vi "Shock&Dyanamics Laboratory - DROPBEAR_June2022_Rev3.vi"() -> ()   [LabVIEW 2019] (continued)
                    n420 = property on="PF Card 29" class="DigNum (strict)"(error in=w420, "DisabledEnum"=w419) -> (error out=w421:errorcluster)  [unwired: 1 in, 1 out]
                    n421 = property on="PF Channel 29" class="DigNum (strict)"(error in=w421, "DisabledEnum"=w419) -> (error out=w422:errorcluster)  [unwired: 1 in, 1 out]
                  }
                  frame True {
                    n422 = stacked-sequence {
                      tunnel: [w427 _] -> w424
                      frame #0 {
                        n423 = property on="PF Condition 29" class="Bool (strict)"() -> (error out=w430:errorcluster, "Value"=w425:bool)  [unwired: 2 in, 1 out]
                        n424 = case shown="True" w425 {
                          tunnel: [T42."Disabled and Grayed Out" ("Disabled") T42."Enabled" ("Disabled")] -> w426
                          frame False {
                          }
                          frame True {
                          }
                        }
                        n425 = property on="PF Chassis 29" class="DigNum (strict)"(error in=w430, "DisabledEnum"=w426) -> (error out=w429:errorcluster)  [unwired: 1 in, 1 out]
                        n426 = property on="PF Card 29" class="DigNum (strict)"(error in=w429, "DisabledEnum"=w426) -> (error out=w428:errorcluster)  [unwired: 1 in, 1 out]
                        n427 = property on="PF Channel 29" class="DigNum (strict)"(error in=w428, "DisabledEnum"=w426) -> (error out=w427:errorcluster)  [unwired: 1 in, 1 out]
                      }
                      frame #1 {
                        n428 = property on="Signal Type 29" class="Enum (strict)"() -> (error out=w435:errorcluster, "Value"=w436:T8)  [unwired: 2 in, 1 out]
                        n429 = case shown="\"Voltage\", Default" w436 {
                          tunnel: [T42."Enabled" ("Disabled") T42."Disabled and Grayed Out" ("Disabled")] -> w434
                          frame "Strain" {
                          }
                          frame "Voltage", Default {
                          }
                        }
                        n430 = property on="SG Pair 29" class="Bool (strict)"(error in=w435, "DisabledEnum"=w434) -> (error out=w433:errorcluster)  [unwired: 1 in, 1 out]
                        n431 = property on="SG Pair Ch 29" class="Enum (strict)"(error in=w433, "DisabledEnum"=w434) -> ()  [unwired: 1 in, 2 out]
                      }
                    }
                  }
                }
                n432 = case shown="False" w208 {
                  tunnel: [w573 T42."Enabled" ("Disabled")] -> w126
                  tunnel: [w576 w577] -> w151
                  frame False {
                    w573 = T42."Disabled and Grayed Out" ("Disabled")
                    n433 = property on="SG Pair 22" class="Bool (strict)"("DisabledEnum"=w573) -> (error out=w572:errorcluster)  [unwired: 2 in, 1 out]
                    n434 = property on="SG Pair Ch 22" class="Enum (strict)"(error in=w572, "DisabledEnum"=w573) -> (error out=w571:errorcluster)  [unwired: 1 in, 1 out]
                    n435 = property on="PF Chassis 22" class="DigNum (strict)"(error in=w571, "DisabledEnum"=w573) -> (error out=w574:errorcluster)  [unwired: 1 in, 1 out]
                    n436 = property on="PF Card 22" class="DigNum (strict)"(error in=w574, "DisabledEnum"=w573) -> (error out=w575:errorcluster)  [unwired: 1 in, 1 out]
                    n437 = property on="PF Channel 22" class="DigNum (strict)"(error in=w575, "DisabledEnum"=w573) -> (error out=w576:errorcluster)  [unwired: 1 in, 1 out]
                  }
                  frame True {
                    n438 = stacked-sequence {
                      tunnel: [w583 _] -> w577
                      frame #0 {
                        n439 = property on="PF Condition 22" class="Bool (strict)"() -> (error out=w580:errorcluster, "Value"=w584:bool)  [unwired: 2 in, 1 out]
                        n440 = case shown="True" w584 {
                          tunnel: [T42."Disabled and Grayed Out" ("Disabled") T42."Enabled" ("Disabled")] -> w579
                          frame False {
                          }
                          frame True {
                          }
                        }
                        n441 = property on="PF Chassis 22" class="DigNum (strict)"(error in=w580, "DisabledEnum"=w579) -> (error out=w581:errorcluster)  [unwired: 1 in, 1 out]
                        n442 = property on="PF Card 22" class="DigNum (strict)"(error in=w581, "DisabledEnum"=w579) -> (error out=w582:errorcluster)  [unwired: 1 in, 1 out]
                        n443 = property on="PF Channel 22" class="DigNum (strict)"(error in=w582, "DisabledEnum"=w579) -> (error out=w583:errorcluster)  [unwired: 1 in, 1 out]
                      }
                      frame #1 {
                        n444 = property on="Signal Type 22" class="Enum (strict)"() -> (error out=w589:errorcluster, "Value"=w590:T8)  [unwired: 2 in, 1 out]
                        n445 = case shown="\"Voltage\", Default" w590 {
                          tunnel: [T42."Enabled" ("Disabled") T42."Disabled and Grayed Out" ("Disabled")] -> w588
                          frame "Strain" {
                          }
                          frame "Voltage", Default {
                          }
                        }
                        n446 = property on="SG Pair 22" class="Bool (strict)"(error in=w589, "DisabledEnum"=w588) -> (error out=w587:errorcluster)  [unwired: 1 in, 1 out]
                        n447 = property on="SG Pair Ch 22" class="Enum (strict)"(error in=w587, "DisabledEnum"=w588) -> ()  [unwired: 1 in, 2 out]
                      }
                    }
                  }
                }
                n448 = case shown="False" w206 {
                  tunnel: [w529 T42."Enabled" ("Disabled")] -> w124
                  tunnel: [w532 w533] -> w135
                  frame False {
                    w529 = T42."Disabled and Grayed Out" ("Disabled")
                    n449 = property on="SG Pair 24" class="Bool (strict)"("DisabledEnum"=w529) -> (error out=w528:errorcluster)  [unwired: 2 in, 1 out]
                    n450 = property on="SG Pair Ch 24" class="Enum (strict)"(error in=w528, "DisabledEnum"=w529) -> (error out=w527:errorcluster)  [unwired: 1 in, 1 out]
                    n451 = property on="PF Chassis 24" class="DigNum (strict)"(error in=w527, "DisabledEnum"=w529) -> (error out=w530:errorcluster)  [unwired: 1 in, 1 out]
                    n452 = property on="PF Card 24" class="DigNum (strict)"(error in=w530, "DisabledEnum"=w529) -> (error out=w531:errorcluster)  [unwired: 1 in, 1 out]
                    n453 = property on="PF Channel 24" class="DigNum (strict)"(error in=w531, "DisabledEnum"=w529) -> (error out=w532:errorcluster)  [unwired: 1 in, 1 out]
                  }
                  frame True {
                    n454 = stacked-sequence {
                      tunnel: [w535 _] -> w533
                      frame #0 {
                        n455 = property on="PF Condition 24" class="Bool (strict)"() -> (error out=w538:errorcluster, "Value"=w540:bool)  [unwired: 2 in, 1 out]
                        n456 = case shown="True" w540 {
                          tunnel: [T42."Disabled and Grayed Out" ("Disabled") T42."Enabled" ("Disabled")] -> w539
                          frame False {
                          }
                          frame True {
                          }
                        }
                        n457 = property on="PF Chassis 24" class="DigNum (strict)"(error in=w538, "DisabledEnum"=w539) -> (error out=w537:errorcluster)  [unwired: 1 in, 1 out]
                        n458 = property on="PF Card 24" class="DigNum (strict)"(error in=w537, "DisabledEnum"=w539) -> (error out=w536:errorcluster)  [unwired: 1 in, 1 out]
                        n459 = property on="PF Channel 24" class="DigNum (strict)"(error in=w536, "DisabledEnum"=w539) -> (error out=w535:errorcluster)  [unwired: 1 in, 1 out]
                      }
                      frame #1 {
                        n460 = property on="Signal Type 24" class="Enum (strict)"() -> (error out=w545:errorcluster, "Value"=w546:T8)  [unwired: 2 in, 1 out]
                        n461 = case shown="\"Voltage\", Default" w546 {
                          tunnel: [T42."Enabled" ("Disabled") T42."Disabled and Grayed Out" ("Disabled")] -> w544
                          frame "Strain" {
                          }
                          frame "Voltage", Default {
                          }
                        }
                        n462 = property on="SG Pair 24" class="Bool (strict)"(error in=w545, "DisabledEnum"=w544) -> (error out=w543:errorcluster)  [unwired: 1 in, 1 out]
                        n463 = property on="SG Pair Ch 24" class="Enum (strict)"(error in=w543, "DisabledEnum"=w544) -> ()  [unwired: 1 in, 2 out]
                      }
                    }
                  }
                }
                n464 = case shown="False" w205 {
                  tunnel: [w507 T42."Enabled" ("Disabled")] -> w115
                  tunnel: [w510 w512] -> w123
                  frame False {
                    w507 = T42."Disabled and Grayed Out" ("Disabled")
                    n465 = property on="SG Pair 25" class="Bool (strict)"("DisabledEnum"=w507) -> (error out=w506:errorcluster)  [unwired: 2 in, 1 out]
                    n466 = property on="SG Pair Ch 25" class="Enum (strict)"(error in=w506, "DisabledEnum"=w507) -> (error out=w505:errorcluster)  [unwired: 1 in, 1 out]
                    n467 = property on="PF Chassis 25" class="DigNum (strict)"(error in=w505, "DisabledEnum"=w507) -> (error out=w508:errorcluster)  [unwired: 1 in, 1 out]
                    n468 = property on="PF Card 25" class="DigNum (strict)"(error in=w508, "DisabledEnum"=w507) -> (error out=w509:errorcluster)  [unwired: 1 in, 1 out]
                    n469 = property on="PF Channel 25" class="DigNum (strict)"(error in=w509, "DisabledEnum"=w507) -> (error out=w510:errorcluster)  [unwired: 1 in, 1 out]
                  }
                  frame True {
                    n470 = stacked-sequence {
                      tunnel: [w513 _] -> w512
                      frame #0 {
                        n471 = property on="PF Condition 25" class="Bool (strict)"() -> (error out=w517:errorcluster, "Value"=w518:bool)  [unwired: 2 in, 1 out]
                        n472 = case shown="True" w518 {
                          tunnel: [T42."Disabled and Grayed Out" ("Disabled") T42."Enabled" ("Disabled")] -> w516
                          frame False {
                          }
                          frame True {
                          }
                        }
                        n473 = property on="PF Chassis 25" class="DigNum (strict)"(error in=w517, "DisabledEnum"=w516) -> (error out=w515:errorcluster)  [unwired: 1 in, 1 out]
                        n474 = property on="PF Card 25" class="DigNum (strict)"(error in=w515, "DisabledEnum"=w516) -> (error out=w514:errorcluster)  [unwired: 1 in, 1 out]
                        n475 = property on="PF Channel 25" class="DigNum (strict)"(error in=w514, "DisabledEnum"=w516) -> (error out=w513:errorcluster)  [unwired: 1 in, 1 out]
                      }
                      frame #1 {
                        n476 = property on="Signal Type 25" class="Enum (strict)"() -> (error out=w523:errorcluster, "Value"=w524:T8)  [unwired: 2 in, 1 out]
                        n477 = case shown="\"Voltage\", Default" w524 {
                          tunnel: [T42."Enabled" ("Disabled") T42."Disabled and Grayed Out" ("Disabled")] -> w522
                          frame "Strain" {
                          }
                          frame "Voltage", Default {
                          }
                        }
                        n478 = property on="SG Pair 25" class="Bool (strict)"(error in=w523, "DisabledEnum"=w522) -> (error out=w521:errorcluster)  [unwired: 1 in, 1 out]
                        n479 = property on="SG Pair Ch 25" class="Enum (strict)"(error in=w521, "DisabledEnum"=w522) -> ()  [unwired: 1 in, 2 out]
                      }
                    }
                  }
                }
                n480 = case shown="False" w200 {
                  tunnel: [w397 T42."Enabled" ("Disabled")] -> w78
                  tunnel: [w400 w402] -> w70
                  frame False {
                    w397 = T42."Disabled and Grayed Out" ("Disabled")
                    n481 = property on="SG Pair 30" class="Bool (strict)"("DisabledEnum"=w397) -> (error out=w396:errorcluster)  [unwired: 2 in, 1 out]
                    n482 = property on="SG Pair Ch 30" class="Enum (strict)"(error in=w396, "DisabledEnum"=w397) -> (error out=w395:errorcluster)  [unwired: 1 in, 1 out]
                    n483 = property on="PF Chassis 30" class="DigNum (strict)"(error in=w395, "DisabledEnum"=w397) -> (error out=w398:errorcluster)  [unwired: 1 in, 1 out]
                    n484 = property on="PF Card 30" class="DigNum (strict)"(error in=w398, "DisabledEnum"=w397) -> (error out=w399:errorcluster)  [unwired: 1 in, 1 out]
                    n485 = property on="PF Channel 30" class="DigNum (strict)"(error in=w399, "DisabledEnum"=w397) -> (error out=w400:errorcluster)  [unwired: 1 in, 1 out]
                  }
                  frame True {
                    n486 = stacked-sequence {
                      tunnel: [w404 _] -> w402
                      frame #0 {
                        n487 = property on="PF Condition 30" class="Bool (strict)"() -> (error out=w407:errorcluster, "Value"=w408:bool)  [unwired: 2 in, 1 out]
                        n488 = case shown="True" w408 {
                          tunnel: [T42."Disabled and Grayed Out" ("Disabled") T42."Enabled" ("Disabled")] -> w403
                          frame False {
                          }
                          frame True {
                          }
                        }
                        n489 = property on="PF Chassis 30" class="DigNum (strict)"(error in=w407, "DisabledEnum"=w403) -> (error out=w406:errorcluster)  [unwired: 1 in, 1 out]
                        n490 = property on="PF Card 30" class="DigNum (strict)"(error in=w406, "DisabledEnum"=w403) -> (error out=w405:errorcluster)  [unwired: 1 in, 1 out]
                        n491 = property on="PF Channel 30" class="DigNum (strict)"(error in=w405, "DisabledEnum"=w403) -> (error out=w404:errorcluster)  [unwired: 1 in, 1 out]
                      }
                      frame #1 {
                        n492 = property on="Signal Type 30" class="Enum (strict)"() -> (error out=w413:errorcluster, "Value"=w414:T8)  [unwired: 2 in, 1 out]
                        n493 = case shown="\"Voltage\", Default" w414 {
                          tunnel: [T42."Enabled" ("Disabled") T42."Disabled and Grayed Out" ("Disabled")] -> w412
                          frame "Strain" {
                          }
                          frame "Voltage", Default {
                          }
                        }
                        n494 = property on="SG Pair 30" class="Bool (strict)"(error in=w413, "DisabledEnum"=w412) -> (error out=w411:errorcluster)  [unwired: 1 in, 1 out]
                        n495 = property on="SG Pair Ch 30" class="Enum (strict)"(error in=w411, "DisabledEnum"=w412) -> ()  [unwired: 1 in, 2 out]
                      }
                    }
                  }
                }
                n496 = case shown="False" w204 {
                  tunnel: [w485 T42."Enabled" ("Disabled")] -> w114
                  tunnel: [w488 w490] -> w106
                  frame False {
                    w485 = T42."Disabled and Grayed Out" ("Disabled")
                    n497 = property on="SG Pair 26" class="Bool (strict)"("DisabledEnum"=w485) -> (error out=w484:errorcluster)  [unwired: 2 in, 1 out]
                    n498 = property on="SG Pair Ch 26" class="Enum (strict)"(error in=w484, "DisabledEnum"=w485) -> (error out=w483:errorcluster)  [unwired: 1 in, 1 out]
                    n499 = property on="PF Chassis 26" class="DigNum (strict)"(error in=w483, "DisabledEnum"=w485) -> (error out=w486:errorcluster)  [unwired: 1 in, 1 out]
                    n500 = property on="PF Card 26" class="DigNum (strict)"(error in=w486, "DisabledEnum"=w485) -> (error out=w487:errorcluster)  [unwired: 1 in, 1 out]
                    n501 = property on="PF Channel 26" class="DigNum (strict)"(error in=w487, "DisabledEnum"=w485) -> (error out=w488:errorcluster)  [unwired: 1 in, 1 out]
                  }
                  frame True {
                    n502 = stacked-sequence {
                      tunnel: [w493 _] -> w490
                      frame #0 {
                        n503 = property on="PF Condition 26" class="Bool (strict)"() -> (error out=w495:errorcluster, "Value"=w496:bool)  [unwired: 2 in, 1 out]
                        n504 = case shown="True" w496 {
                          tunnel: [T42."Disabled and Grayed Out" ("Disabled") T42."Enabled" ("Disabled")] -> w494
                          frame False {
                          }
                          frame True {
                          }
                        }
                        n505 = property on="PF Chassis 26" class="DigNum (strict)"(error in=w495, "DisabledEnum"=w494) -> (error out=w491:errorcluster)  [unwired: 1 in, 1 out]
                        n506 = property on="PF Card 26" class="DigNum (strict)"(error in=w491, "DisabledEnum"=w494) -> (error out=w492:errorcluster)  [unwired: 1 in, 1 out]
                        n507 = property on="PF Channel 26" class="DigNum (strict)"(error in=w492, "DisabledEnum"=w494) -> (error out=w493:errorcluster)  [unwired: 1 in, 1 out]
                      }
                      frame #1 {
                        n508 = property on="Signal Type 26" class="Enum (strict)"() -> (error out=w501:errorcluster, "Value"=w502:T8)  [unwired: 2 in, 1 out]
                        n509 = case shown="\"Voltage\", Default" w502 {
                          tunnel: [T42."Enabled" ("Disabled") T42."Disabled and Grayed Out" ("Disabled")] -> w500
                          frame "Strain" {
                          }
                          frame "Voltage", Default {
                          }
                        }
                        n510 = property on="SG Pair 26" class="Bool (strict)"(error in=w501, "DisabledEnum"=w500) -> (error out=w499:errorcluster)  [unwired: 1 in, 1 out]
                        n511 = property on="SG Pair Ch 26" class="Enum (strict)"(error in=w499, "DisabledEnum"=w500) -> ()  [unwired: 1 in, 2 out]
                      }
                    }
                  }
                }
                n512 = case shown="False" w203 {
                  tunnel: [w463 T42."Enabled" ("Disabled")] -> w97
                  tunnel: [w466 w468] -> w105
                  frame False {
                    w463 = T42."Disabled and Grayed Out" ("Disabled")
                    n513 = property on="SG Pair 27" class="Bool (strict)"("DisabledEnum"=w463) -> (error out=w462:errorcluster)  [unwired: 2 in, 1 out]
                    n514 = property on="SG Pair Ch 27" class="Enum (strict)"(error in=w462, "DisabledEnum"=w463) -> (error out=w461:errorcluster)  [unwired: 1 in, 1 out]
                    n515 = property on="PF Chassis 27" class="DigNum (strict)"(error in=w461, "DisabledEnum"=w463) -> (error out=w464:errorcluster)  [unwired: 1 in, 1 out]
                    n516 = property on="PF Card 27" class="DigNum (strict)"(error in=w464, "DisabledEnum"=w463) -> (error out=w465:errorcluster)  [unwired: 1 in, 1 out]
                    n517 = property on="PF Channel 27" class="DigNum (strict)"(error in=w465, "DisabledEnum"=w463) -> (error out=w466:errorcluster)  [unwired: 1 in, 1 out]
                  }
                  frame True {
                    n518 = stacked-sequence {
                      tunnel: [w469 _] -> w468
                      frame #0 {
                        n519 = property on="PF Condition 27" class="Bool (strict)"() -> (error out=w473:errorcluster, "Value"=w474:bool)  [unwired: 2 in, 1 out]
                        n520 = case shown="True" w474 {
                          tunnel: [T42."Disabled and Grayed Out" ("Disabled") T42."Enabled" ("Disabled")] -> w472
                          frame False {
                          }
                          frame True {
                          }
                        }
                        n521 = property on="PF Chassis 27" class="DigNum (strict)"(error in=w473, "DisabledEnum"=w472) -> (error out=w471:errorcluster)  [unwired: 1 in, 1 out]
                        n522 = property on="PF Card 27" class="DigNum (strict)"(error in=w471, "DisabledEnum"=w472) -> (error out=w470:errorcluster)  [unwired: 1 in, 1 out]
                        n523 = property on="PF Channel 27" class="DigNum (strict)"(error in=w470, "DisabledEnum"=w472) -> (error out=w469:errorcluster)  [unwired: 1 in, 1 out]
                      }
                      frame #1 {
                        n524 = property on="Signal Type 27" class="Enum (strict)"() -> (error out=w479:errorcluster, "Value"=w480:T8)  [unwired: 2 in, 1 out]
                        n525 = case shown="\"Voltage\", Default" w480 {
                          tunnel: [T42."Enabled" ("Disabled") T42."Disabled and Grayed Out" ("Disabled")] -> w478
                          frame "Strain" {
                          }
                          frame "Voltage", Default {
                          }
                        }
                        n526 = property on="SG Pair 27" class="Bool (strict)"(error in=w479, "DisabledEnum"=w478) -> (error out=w477:errorcluster)  [unwired: 1 in, 1 out]
                        n527 = property on="SG Pair Ch 27" class="Enum (strict)"(error in=w477, "DisabledEnum"=w478) -> ()  [unwired: 1 in, 2 out]
                      }
                    }
                  }
                }
                n528 = case shown="False" w202 {
                  tunnel: [w441 T42."Enabled" ("Disabled")] -> w96
                  tunnel: [w444 w445] -> w88
                  frame False {
                    w441 = T42."Disabled and Grayed Out" ("Disabled")
                    n529 = property on="SG Pair 28" class="Bool (strict)"("DisabledEnum"=w441) -> (error out=w440:errorcluster)  [unwired: 2 in, 1 out]
                    n530 = property on="SG Pair Ch 28" class="Enum (strict)"(error in=w440, "DisabledEnum"=w441) -> (error out=w439:errorcluster)  [unwired: 1 in, 1 out]
                    n531 = property on="PF Chassis 28" class="DigNum (strict)"(error in=w439, "DisabledEnum"=w441) -> (error out=w442:errorcluster)  [unwired: 1 in, 1 out]
                    n532 = property on="PF Card 28" class="DigNum (strict)"(error in=w442, "DisabledEnum"=w441) -> (error out=w443:errorcluster)  [unwired: 1 in, 1 out]
                    n533 = property on="PF Channel 28" class="DigNum (strict)"(error in=w443, "DisabledEnum"=w441) -> (error out=w444:errorcluster)  [unwired: 1 in, 1 out]
                  }
                  frame True {
                    n534 = stacked-sequence {
                      tunnel: [w447 _] -> w445
                      frame #0 {
                        n535 = property on="PF Condition 28" class="Bool (strict)"() -> (error out=w450:errorcluster, "Value"=w451:bool)  [unwired: 2 in, 1 out]
                        n536 = case shown="True" w451 {
                          tunnel: [T42."Disabled and Grayed Out" ("Disabled") T42."Enabled" ("Disabled")] -> w452
                          frame False {
                          }
                          frame True {
                          }
                        }
                        n537 = property on="PF Chassis 28" class="DigNum (strict)"(error in=w450, "DisabledEnum"=w452) -> (error out=w449:errorcluster)  [unwired: 1 in, 1 out]
                        n538 = property on="PF Card 28" class="DigNum (strict)"(error in=w449, "DisabledEnum"=w452) -> (error out=w448:errorcluster)  [unwired: 1 in, 1 out]
                        n539 = property on="PF Channel 28" class="DigNum (strict)"(error in=w448, "DisabledEnum"=w452) -> (error out=w447:errorcluster)  [unwired: 1 in, 1 out]
                      }
                      frame #1 {
                        n540 = property on="Signal Type 28" class="Enum (strict)"() -> (error out=w457:errorcluster, "Value"=w458:T8)  [unwired: 2 in, 1 out]
                        n541 = case shown="\"Voltage\", Default" w458 {
                          tunnel: [T42."Enabled" ("Disabled") T42."Disabled and Grayed Out" ("Disabled")] -> w456
                          frame "Strain" {
                          }
                          frame "Voltage", Default {
                          }
                        }
                        n542 = property on="SG Pair 28" class="Bool (strict)"(error in=w457, "DisabledEnum"=w456) -> (error out=w455:errorcluster)  [unwired: 1 in, 1 out]
                        n543 = property on="SG Pair Ch 28" class="Enum (strict)"(error in=w455, "DisabledEnum"=w456) -> ()  [unwired: 1 in, 2 out]
                      }
                    }
                  }
                }
                n544 = case shown="False" w199 {
                  tunnel: [w375 T42."Enabled" ("Disabled")] -> w69
                  tunnel: [w378 w379] -> w61
                  frame False {
                    w375 = T42."Disabled and Grayed Out" ("Disabled")
                    n545 = property on="SG Pair 31" class="Bool (strict)"("DisabledEnum"=w375) -> (error out=w374:errorcluster)  [unwired: 2 in, 1 out]
                    n546 = property on="SG Pair Ch 31" class="Enum (strict)"(error in=w374, "DisabledEnum"=w375) -> (error out=w373:errorcluster)  [unwired: 1 in, 1 out]
                    n547 = property on="PF Chassis 31" class="DigNum (strict)"(error in=w373, "DisabledEnum"=w375) -> (error out=w376:errorcluster)  [unwired: 1 in, 1 out]
                    n548 = property on="PF Card 31" class="DigNum (strict)"(error in=w376, "DisabledEnum"=w375) -> (error out=w377:errorcluster)  [unwired: 1 in, 1 out]
                    n549 = property on="PF Channel 31" class="DigNum (strict)"(error in=w377, "DisabledEnum"=w375) -> (error out=w378:errorcluster)  [unwired: 1 in, 1 out]
                  }
                  frame True {
                    n550 = stacked-sequence {
                      tunnel: [w382 _] -> w379
                      frame #0 {
                        n551 = property on="PF Condition 31" class="Bool (strict)"() -> (error out=w385:errorcluster, "Value"=w386:bool)  [unwired: 2 in, 1 out]
                        n552 = case shown="True" w386 {
                          tunnel: [T42."Disabled and Grayed Out" ("Disabled") T42."Enabled" ("Disabled")] -> w381
                          frame False {
                          }
                          frame True {
                          }
                        }
                        n553 = property on="PF Chassis 31" class="DigNum (strict)"(error in=w385, "DisabledEnum"=w381) -> (error out=w384:errorcluster)  [unwired: 1 in, 1 out]
                        n554 = property on="PF Card 31" class="DigNum (strict)"(error in=w384, "DisabledEnum"=w381) -> (error out=w383:errorcluster)  [unwired: 1 in, 1 out]
                        n555 = property on="PF Channel 31" class="DigNum (strict)"(error in=w383, "DisabledEnum"=w381) -> (error out=w382:errorcluster)  [unwired: 1 in, 1 out]
                      }
                      frame #1 {
                        n556 = property on="Signal Type 31" class="Enum (strict)"() -> (error out=w392:errorcluster, "Value"=w391:T8)  [unwired: 2 in, 1 out]
                        n557 = case shown="\"Voltage\", Default" w391 {
                          tunnel: [T42."Enabled" ("Disabled") T42."Disabled and Grayed Out" ("Disabled")] -> w390
                          frame "Strain" {
                          }
                          frame "Voltage", Default {
                          }
                        }
                        n558 = property on="SG Pair 31" class="Bool (strict)"(error in=w392, "DisabledEnum"=w390) -> (error out=w389:errorcluster)  [unwired: 1 in, 1 out]
                        n559 = property on="SG Pair Ch 31" class="Enum (strict)"(error in=w389, "DisabledEnum"=w390) -> ()  [unwired: 1 in, 2 out]
                      }
                    }
                  }
                }
                n560 = property on="Signal Type 24" class="Enum (strict)"(error in=w135, "DisabledEnum"=w124) -> (error out=w134:errorcluster)  [unwired: 1 in, 1 out]
                n561 = property on="Signal Type 23" class="Enum (strict)"(error in=w143, "DisabledEnum"=w125) -> (error out=w142:errorcluster)  [unwired: 1 in, 1 out]
                n562 = property on="Signal Type 19" class="Enum (strict)"(error in=w169, "DisabledEnum"=w177) -> (error out=w170:errorcluster)  [unwired: 1 in, 1 out]
                n563 = property on="Signal Type 21" class="Enum (strict)"(error in=w159, "DisabledEnum"=w127) -> (error out=w158:errorcluster)  [unwired: 1 in, 1 out]
                n564 = property on="Signal Type 18" class="Enum (strict)"(error in=w186, "DisabledEnum"=w178) -> (error out=w185:errorcluster)  [unwired: 1 in, 1 out]
                n565 = property on="Signal Type 22" class="Enum (strict)"(error in=w151, "DisabledEnum"=w126) -> (error out=w150:errorcluster)  [unwired: 1 in, 1 out]
                n566 = property on="Signal Type 20" class="Enum (strict)"(error in=w168, "DisabledEnum"=w160) -> (error out=w167:errorcluster)  [unwired: 1 in, 1 out]
                n567 = property on="Physical Channel Ch 24" class="DAQmxName"(error in=w134, "DisabledEnum"=w124) -> (error out=w133:errorcluster)  [unwired: 1 in, 1 out]
                n568 = property on="Physical Channel Ch 23" class="DAQmxName"(error in=w142, "DisabledEnum"=w125) -> (error out=w141:errorcluster)  [unwired: 1 in, 1 out]
                n569 = property on="Physical Channel Ch 19" class="DAQmxName"(error in=w170, "DisabledEnum"=w177) -> (error out=w171:errorcluster)  [unwired: 1 in, 1 out]
                n570 = property on="Physical Channel Ch 18" class="DAQmxName"(error in=w185, "DisabledEnum"=w178) -> (error out=w184:errorcluster)  [unwired: 1 in, 1 out]
                n571 = property on="Physical Channel Ch 21" class="DAQmxName"(error in=w158, "DisabledEnum"=w127) -> (error out=w157:errorcluster)  [unwired: 1 in, 1 out]
                n572 = property on="Physical Channel Ch 22" class="DAQmxName"(error in=w150, "DisabledEnum"=w126) -> (error out=w149:errorcluster)  [unwired: 1 in, 1 out]
                n573 = property on="Physical Channel Ch 20" class="DAQmxName"(error in=w167, "DisabledEnum"=w160) -> (error out=w166:errorcluster)  [unwired: 1 in, 1 out]
                n574 = property on="Signal Type 1" class="Enum (strict)"(error in=w335, "DisabledEnum"=w365) -> (error out=w367:errorcluster)  [unwired: 1 in, 1 out]
                n575 = property on="Signal Type 17" class="Enum (strict)"(error in=w195, "DisabledEnum"=w187) -> (error out=w194:errorcluster)  [unwired: 1 in, 1 out]
                n576 = property on="Signal Type 2" class="Enum (strict)"(error in=w334, "DisabledEnum"=w356) -> (error out=w358:errorcluster)  [unwired: 1 in, 1 out]
                n577 = property on="Signal Type 4" class="Enum (strict)"(error in=w332, "DisabledEnum"=w340) -> (error out=w342:errorcluster)  [unwired: 1 in, 1 out]
                n578 = property on="Signal Type 5" class="Enum (strict)"(error in=w323, "DisabledEnum"=w325) -> (error out=w327:errorcluster)  [unwired: 1 in, 1 out]
                n579 = property on="Signal Type 6" class="Enum (strict)"(error in=w313, "DisabledEnum"=w315) -> (error out=w317:errorcluster)  [unwired: 1 in, 1 out]
                n580 = property on="Signal Type 12" class="Enum (strict)"(error in=w254, "DisabledEnum"=w256) -> (error out=w258:errorcluster)  [unwired: 1 in, 1 out]
                n581 = property on="Signal Type 13" class="Enum (strict)"(error in=w245, "DisabledEnum"=w247) -> (error out=w249:errorcluster)  [unwired: 1 in, 1 out]
                n582 = property on="Signal Type 15" class="Enum (strict)"(error in=w227, "DisabledEnum"=w229) -> (error out=w231:errorcluster)  [unwired: 1 in, 1 out]
                n583 = property on="Signal Type 7" class="Enum (strict)"(error in=w304, "DisabledEnum"=w306) -> (error out=w308:errorcluster)  [unwired: 1 in, 1 out]
                n584 = property on="Signal Type 11" class="Enum (strict)"(error in=w263, "DisabledEnum"=w265) -> (error out=w267:errorcluster)  [unwired: 1 in, 1 out]
                n585 = property on="Signal Type 14" class="Enum (strict)"(error in=w236, "DisabledEnum"=w238) -> (error out=w240:errorcluster)  [unwired: 1 in, 1 out]
                n586 = property on="Signal Type 16" class="Enum (strict)"(error in=w198, "DisabledEnum"=w197) -> (error out=w196:errorcluster)  [unwired: 1 in, 1 out]
                n587 = property on="Signal Type 8" class="Enum (strict)"(error in=w293, "DisabledEnum"=w295) -> (error out=w297:errorcluster)  [unwired: 1 in, 1 out]
                n588 = property on="Signal Type 9" class="Enum (strict)"(error in=w284, "DisabledEnum"=w286) -> (error out=w288:errorcluster)  [unwired: 1 in, 1 out]
                n589 = property on="Signal Type 10" class="Enum (strict)"(error in=w275, "DisabledEnum"=w277) -> (error out=w279:errorcluster)  [unwired: 1 in, 1 out]
                n590 = property on="Signal Type 3" class="Enum (strict)"(error in=w333, "DisabledEnum"=w348) -> (error out=w350:errorcluster)  [unwired: 1 in, 1 out]
                n591 = property on="Name Ch 24" class="Str"(error in=w133, "DisabledEnum"=w124) -> (error out=w132:errorcluster)  [unwired: 1 in, 1 out]
                n592 = property on="Name Ch 23" class="Str"(error in=w141, "DisabledEnum"=w125) -> (error out=w140:errorcluster)  [unwired: 1 in, 1 out]
                n593 = property on="Name Ch 19" class="Str"(error in=w171, "DisabledEnum"=w177) -> (error out=w172:errorcluster)  [unwired: 1 in, 1 out]
                n594 = property on="Name Ch 18" class="Str"(error in=w184, "DisabledEnum"=w178) -> (error out=w183:errorcluster)  [unwired: 1 in, 1 out]
                n595 = property on="Name Ch 21" class="Str"(error in=w157, "DisabledEnum"=w127) -> (error out=w156:errorcluster)  [unwired: 1 in, 1 out]
                n596 = property on="Name Ch 22" class="Str"(error in=w149, "DisabledEnum"=w126) -> (error out=w148:errorcluster)  [unwired: 1 in, 1 out]
                n597 = property on="Name Ch 20" class="Str"(error in=w166, "DisabledEnum"=w160) -> (error out=w165:errorcluster)  [unwired: 1 in, 1 out]
                n598 = property on="Signal Type 30" class="Enum (strict)"(error in=w70, "DisabledEnum"=w78) -> (error out=w71:errorcluster)  [unwired: 1 in, 1 out]
                n599 = property on="Physical Channel Ch 1" class="DAQmxName"(error in=w367, "DisabledEnum"=w365) -> (error out=w371:errorcluster)  [unwired: 1 in, 1 out]
                n600 = property on="Physical Channel Ch 17" class="DAQmxName"(error in=w194, "DisabledEnum"=w187) -> (error out=w193:errorcluster)  [unwired: 1 in, 1 out]
                n601 = property on="Signal Type 25" class="Enum (strict)"(error in=w123, "DisabledEnum"=w115) -> (error out=w122:errorcluster)  [unwired: 1 in, 1 out]
                n602 = property on="Signal Type 26" class="Enum (strict)"(error in=w106, "DisabledEnum"=w114) -> (error out=w107:errorcluster)  [unwired: 1 in, 1 out]
                n603 = property on="Signal Type 29" class="Enum (strict)"(error in=w79, "DisabledEnum"=w87) -> (error out=w80:errorcluster)  [unwired: 1 in, 1 out]
                n604 = property on="Physical Channel Ch 2" class="DAQmxName"(error in=w358, "DisabledEnum"=w356) -> (error out=w362:errorcluster)  [unwired: 1 in, 1 out]
                n605 = property on="Signal Type 28" class="Enum (strict)"(error in=w88, "DisabledEnum"=w96) -> (error out=w89:errorcluster)  [unwired: 1 in, 1 out]
                n606 = property on="Signal Type 27" class="Enum (strict)"(error in=w105, "DisabledEnum"=w97) -> (error out=w104:errorcluster)  [unwired: 1 in, 1 out]
                n607 = property on="Physical Channel Ch 4" class="DAQmxName"(error in=w342, "DisabledEnum"=w340) -> (error out=w346:errorcluster)  [unwired: 1 in, 1 out]
                n608 = property on="Physical Channel Ch 5" class="DAQmxName"(error in=w327, "DisabledEnum"=w325) -> (error out=w331:errorcluster)  [unwired: 1 in, 1 out]
                n609 = property on="Signal Type 31" class="Enum (strict)"(error in=w61, "DisabledEnum"=w69) -> (error out=w62:errorcluster)  [unwired: 1 in, 1 out]
                n610 = property on="Physical Channels Ch 6" class="DAQmxName"(error in=w317, "DisabledEnum"=w315) -> (error out=w321:errorcluster)  [unwired: 1 in, 1 out]
                n611 = property on="Physical Channel Ch 12" class="DAQmxName"(error in=w258, "DisabledEnum"=w256) -> (error out=w262:errorcluster)  [unwired: 1 in, 1 out]
                n612 = property on="Physical Channel Ch 13" class="DAQmxName"(error in=w249, "DisabledEnum"=w247) -> (error out=w253:errorcluster)  [unwired: 1 in, 1 out]
                n613 = property on="Physical Channel Ch 15" class="DAQmxName"(error in=w231, "DisabledEnum"=w229) -> (error out=w235:errorcluster)  [unwired: 1 in, 1 out]
                n614 = property on="Physical Channel Ch 7" class="DAQmxName"(error in=w308, "DisabledEnum"=w306) -> (error out=w312:errorcluster)  [unwired: 1 in, 1 out]
                n615 = property on="Physical Channel Ch 11" class="DAQmxName"(error in=w267, "DisabledEnum"=w265) -> (error out=w271:errorcluster)  [unwired: 1 in, 1 out]
                n616 = property on="Physical Channel Ch 14" class="DAQmxName"(error in=w240, "DisabledEnum"=w238) -> (error out=w244:errorcluster)  [unwired: 1 in, 1 out]
                n617 = property on="Physical Channel Ch 8" class="DAQmxName"(error in=w297, "DisabledEnum"=w295) -> (error out=w301:errorcluster)  [unwired: 1 in, 1 out]
                n618 = property on="Physical Channel Ch 9" class="DAQmxName"(error in=w288, "DisabledEnum"=w286) -> (error out=w292:errorcluster)  [unwired: 1 in, 1 out]
                n619 = property on="Physical Channel Ch 10" class="DAQmxName"(error in=w279, "DisabledEnum"=w277) -> (error out=w283:errorcluster)  [unwired: 1 in, 1 out]
                n620 = property on="Sens Fac 24" class="Enum (strict)"(error in=w132, "DisabledEnum"=w124) -> (error out=w131:errorcluster)  [unwired: 1 in, 1 out]
                n621 = property on="Physical Channel Ch 16" class="DAQmxName"(error in=w196, "DisabledEnum"=w197) -> (error out=w220:errorcluster)  [unwired: 1 in, 1 out]
                n622 = property on="Sens Fac 21" class="Enum (strict)"(error in=w156, "DisabledEnum"=w127) -> (error out=w155:errorcluster)  [unwired: 1 in, 1 out]
                n623 = property on="Sens Fac 23" class="Enum (strict)"(error in=w140, "DisabledEnum"=w125) -> (error out=w139:errorcluster)  [unwired: 1 in, 1 out]
                n624 = property on="Sens Fac 22" class="Enum (strict)"(error in=w148, "DisabledEnum"=w126) -> (error out=w147:errorcluster)  [unwired: 1 in, 1 out]
                n625 = property on="Physical Channels Ch 3" class="DAQmxName"(error in=w350, "DisabledEnum"=w348) -> (error out=w354:errorcluster)  [unwired: 1 in, 1 out]
                n626 = property on="Sens Fac 18" class="Enum (strict)"(error in=w183, "DisabledEnum"=w178) -> (error out=w182:errorcluster)  [unwired: 1 in, 1 out]
                n627 = property on="Sens Fac 20" class="Enum (strict)"(error in=w165, "DisabledEnum"=w160) -> (error out=w164:errorcluster)  [unwired: 1 in, 1 out]
                n628 = property on="Sens Fac 19" class="Enum (strict)"(error in=w172, "DisabledEnum"=w177) -> (error out=w173:errorcluster)  [unwired: 1 in, 1 out]
                n629 = property on="Physical Channel Ch 30" class="DAQmxName"(error in=w71, "DisabledEnum"=w78) -> (error out=w72:errorcluster)  [unwired: 1 in, 1 out]
                n630 = property on="Physical Channel Ch 25" class="DAQmxName"(error in=w122, "DisabledEnum"=w115) -> (error out=w121:errorcluster)  [unwired: 1 in, 1 out]
                n631 = property on="Physical Channel Ch 29" class="DAQmxName"(error in=w80, "DisabledEnum"=w87) -> (error out=w81:errorcluster)  [unwired: 1 in, 1 out]
                n632 = property on="Sensitivity 24" class="DigNum (strict)"(error in=w131, "DisabledEnum"=w124) -> (error out=w130:errorcluster)  [unwired: 1 in, 1 out]
                n633 = property on="Physical Channel Ch 28" class="DAQmxName"(error in=w89, "DisabledEnum"=w96) -> (error out=w90:errorcluster)  [unwired: 1 in, 1 out]
                n634 = property on="Sensitivity 22" class="DigNum (strict)"(error in=w147, "DisabledEnum"=w126) -> (error out=w146:errorcluster)  [unwired: 1 in, 1 out]
                n635 = property on="Sensitivity 23" class="DigNum (strict)"(error in=w139, "DisabledEnum"=w125) -> (error out=w138:errorcluster)  [unwired: 1 in, 1 out]
                n636 = property on="Sensitivity 18" class="DigNum (strict)"(error in=w182, "DisabledEnum"=w178) -> (error out=w181:errorcluster)  [unwired: 1 in, 1 out]
                n637 = property on="Sensitivity 21" class="DigNum (strict)"(error in=w155, "DisabledEnum"=w127) -> (error out=w154:errorcluster)  [unwired: 1 in, 1 out]
                n638 = property on="Physical Channel Ch 31" class="DAQmxName"(error in=w62, "DisabledEnum"=w69) -> (error out=w63:errorcluster)  [unwired: 1 in, 1 out]
                n639 = property on="Physical Channel Ch 26" class="DAQmxName"(error in=w107, "DisabledEnum"=w114) -> (error out=w108:errorcluster)  [unwired: 1 in, 1 out]
                n640 = property on="Name Ch 17" class="Str"(error in=w193, "DisabledEnum"=w187) -> (error out=w192:errorcluster)  [unwired: 1 in, 1 out]
